vi "Init Data.vi"(8 "error in (no error)":errorcluster, 10 "Data Object":refnum<class "Factory Plugin Framework.lvclass">, 11 "Measurement Interface in":refnum<class "Measurement Interface.lvclass">) -> (0 "error out":errorcluster, 3 "Measurement Interface out":refnum<class "Measurement Interface.lvclass">)   [LabVIEW 2018, in "Measurement Interface.lvlib" / "Measurement Interface.lvclass"]
uses:
  Measurement Interface.lvclass
  Plugins/FPF.lvlibp/Factory Plugin Framework.lvclass
  Measurement Interface.lvclass/Measurement Interface.ctl
  Active Sequence File/Read Active Sequence File.vi
  Engine Reference/Read Engine Reference.vi
  Measurement Parameters/Read Measurement Parameters.vi
  Default Steps Database/Read Default Steps Database.vi
  Public Methods/Sequence Reference/Read Sequence Reference.vi
  Measurement Name/Read Measurement Name.vi
  Sequence Call Step/Read Sequence Call Step Dictionary.vi
  Measurement Definition Entry/Read Measurement Definition Entry.vi
  Test Group Manager/Read Test Group Manager.vi
  Active Sequence File/Write Active Sequence File.vi
  Engine Reference/Write Engine Reference.vi
  Measurement Parameters/Write Measurement Parameters.vi
  Default Steps Database/Write Default Steps Database.vi
  Public Methods/Sequence Reference/Write Sequence Reference.vi
  Measurement Name/Write Measurement Name.vi
  Sequence Call Step/Write Sequence Call Step Dictionary.vi
  Measurement Definition Entry/Write Measurement Definition Entry.vi
  Test Group Manager/Write Test Group Manager.vi
  Plugins/String Database.lvlibp/String Database.lvclass
  Plugins/Sequence Call Step Dictionary.lvlibp/Sequence Call Step Dictionary.lvclass
  Plugins/Test Group Manager.lvlibp/Test Group Manager.lvclass
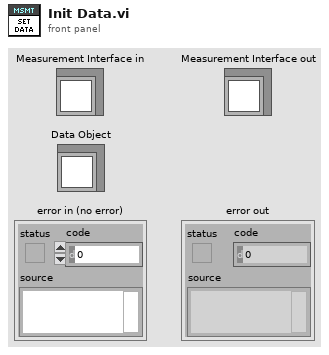
[diagram p1: front panel]
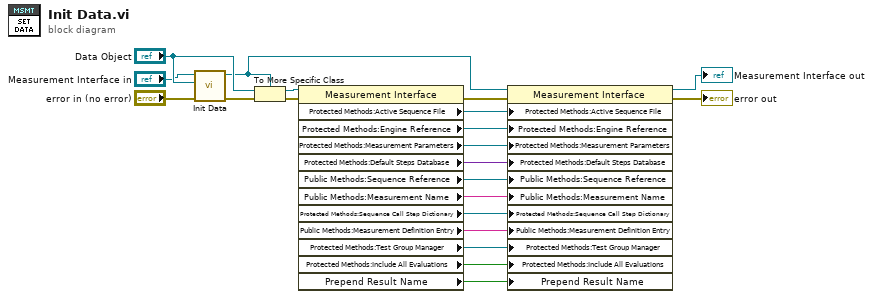
[diagram p0: block diagram]
diagram:
  n1 = call-parent "Init Data.vi"("error in (no error)"="error in (no error)", "Data Object"="Data Object", "Factory Plugin Framework in"="Measurement Interface in") -> ("error out"=w21:errorcluster, "Factory Plugin Framework out"=w9:refnum<class "Measurement Interface.lvclass">)  [unwired: 7 in]
  n2 = To More Specific Class(target class=w9, reference="Data Object", error in=w21) -> (specific class reference=w11:refnum<class "Measurement Interface.lvclass">, error out=w19:errorcluster)
  n3 = property class="Measurement Interface"(reference=w11, error in=w19) -> (error out=w18:errorcluster, "Protected Methods:Active Sequence File"=w15:refnum<k7>, "Protected Methods:Engine Reference"=w14:refnum<k7>, "Protected Methods:Measurement Parameters"=w13:refnum<class "String Database.lvclass">, "Protected Methods:Default Steps Database"=w8:variant, "Public Methods:Sequence Reference"=w7:refnum<k7>, "Public Methods:Measurement Name"=w6:string, "Protected Methods:Sequence Call Step Dictionary"=w5:refnum<class "Sequence Call Step Dictionary.lvclass">, "Public Methods:Measurement Definition Entry"=w4:string, "Protected Methods:Test Group Manager"=w3:refnum<data-value>, "Protected Methods:Include All Evaluations"=w2:bool, "Prepend Result Name"=w1:bool)  [unwired: 1 out]
  n4 = property class="Measurement Interface"(reference=w9, error in=w18, "Protected Methods:Active Sequence File"=w15, "Protected Methods:Engine Reference"=w14, "Protected Methods:Measurement Parameters"=w13, "Protected Methods:Default Steps Database"=w8, "Public Methods:Sequence Reference"=w7, "Public Methods:Measurement Name"=w6, "Protected Methods:Sequence Call Step Dictionary"=w5, "Public Methods:Measurement Definition Entry"=w4, "Protected Methods:Test Group Manager"=w3, "Protected Methods:Include All Evaluations"=w2, "Prepend Result Name"=w1) -> (reference out=→"Measurement Interface out":refnum<class "Measurement Interface.lvclass">, error out=→"error out":errorcluster)
